vi "_Destroy.vi"(8 "error in (no error)":errorcluster, 11 "LCD Retarder in":refnum<class "LCD Retarder.lvclass">) -> (0 "error out":errorcluster)   [LabVIEW 2017, in "LCD Retarder.lvclass"]
uses:
  LCD Retarder.lvclass
  LCD Retarder.lvclass/LCD Retarder.ctl
  Utility Classes/Readable/Readable.lvclass
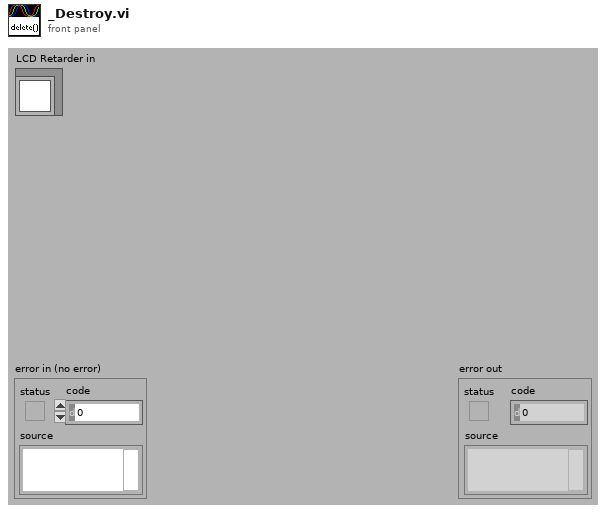
[diagram p1: front panel]
types:
  T1 = cluster{"Device Handle":u32, "Pipe 0 Handle":u32, "Pipe 1 Handle":u32}[]
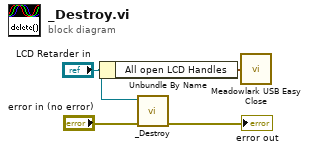
[diagram p0: block diagram]
diagram:
  n1 = Unbundle By Name("LCD Retarder in") -> ("All open LCD Handles"=w1:T1)
  n2 = call-parent "_Destroy.vi"("error in (no error)"="error in (no error)", "Instrument in"="LCD Retarder in") -> ("error out"=→"error out":errorcluster)  [unwired: 9 out]
  n3 = call "Meadowlark USB Easy Close.vi"("USB Device and Pipes Array"=w1) -> ()
